vi "LEP_RV_Show_UV.vi"   [LabVIEW 2011]
types:
  T1 = enum16{"Normal", "Minimized", "Maximized", "Hidden", "Locked"}
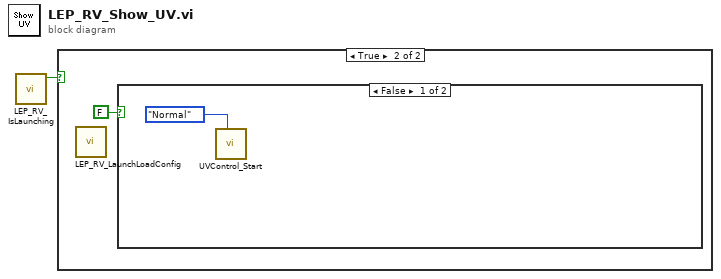
[diagram p0: block diagram]
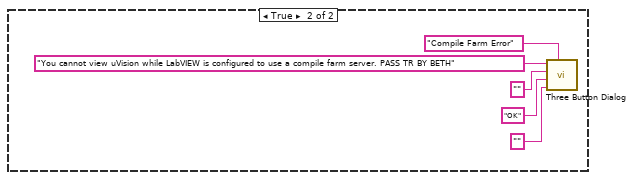
[diagram p3: hidden frame]
diagram:
  n1 = call "LEP_RV_IsLaunching.vi"() -> ("not in memory"=w1:bool)  [unwired: 11 in]
  n2 = case shown="True" w1 {
    frame False {
    }
    frame True {
      n3 = call "LEP_RV_LaunchLoadConfig.vi"() -> ()  [unwired: 8 in, 8 out]
      n4 = case shown="False" FALSE {
        frame False {
          n5 = call "UVControl_Start.vi"("Mode"=T1."Normal") -> ()  [unwired: 8 in, 3 out]
        }
        frame True {
          n6 = call <vilib>:"Three Button Dialog.vi"("Window Title (\"\")"="Compile Farm Error" ("Window Title (\"\")"), "Right Button Text (\"Cancel\")"="" ("Right Button Text (\"Cancel\")"), "Center Button Text (\"No\")"="OK" ("Center Button Text (\"No\")"), "Left Button Text (\"Yes\")"="" ("Left Button Text (\"Yes\")"), "message"="You cannot view uVision while LabVIEW is configured to use a compile farm server. PASS TR BY BETH") -> ()  [unwired: 6 in, 1 out]
        }
      }
    }
  }
